vi "Send Set Loop Period.vi"(8 "error in (no error)":errorcluster, 10 "Loop Period in ms (10)":u32=10, 11 "Message Queue in":refnum<queue>) -> (0 "error out":errorcluster, 3 "Message Queue out":refnum<queue>)   [LabVIEW 2024, in "PID Loop.lvlib" / "Set Loop Period.lvclass"]
uses:
  Set Loop Period.lvclass
  Set Loop Period.lvclass/Set Loop Period.ctl
  C:/Users/uspoaotto/OneDrive - Oregon Tool/Desktop/working copies/helperLoop/src/OOQMH/Message/Message.lvclass
  C:/Users/uspoaotto/OneDrive - Oregon Tool/Desktop/working copies/helperLoop/src/PID Loop/Set Loop Period/Set Loop Period.lvclass
  OOQMH/Message/Message.lvclass
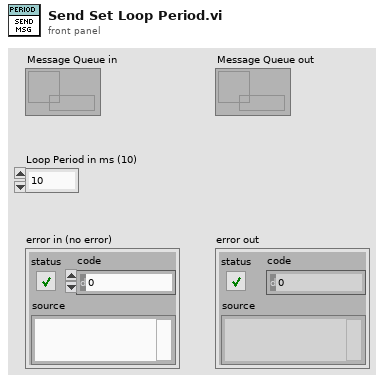
[diagram p1: front panel]
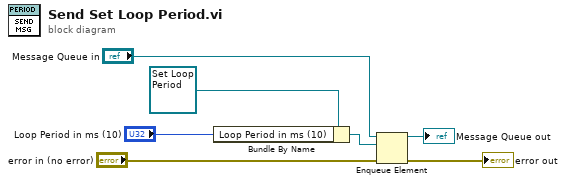
[diagram p0: block diagram]
diagram:
  n1 = Bundle By Name(cluster=refnum<class "Set Loop Period.lvclass"> refnum ("PID Loop.lvlib:Set Loop Period.lvclass"), "Loop Period in ms (10)"="Loop Period in ms (10)") -> (w3:refnum<class "Set Loop Period.lvclass">)
  n2 = Enqueue Element(queue="Message Queue in", element=w3, error in (no error)="error in (no error)") -> (queue out=→"Message Queue out":refnum<queue>, error out=→"error out":errorcluster)  [unwired: 1 in, 1 out]
